vi "MCCPMTzero.vi"(8 "error in (no error)":errorcluster, 11 "MCCPMT in":refnum<class "MCCPMT.lvclass">) -> (0 "error out":errorcluster, 3 "MCCPMT out":refnum<class "MCCPMT.lvclass">)   [LabVIEW 2012, in "MCCPMT.lvclass"]
uses:
  MCCPMT.lvclass
  MCCPMT.lvclass/MCCPMT.ctl
  <vilib>/ULx/Create Channel.llb/ULx Create Channel (AO-Voltage-Basic).vi
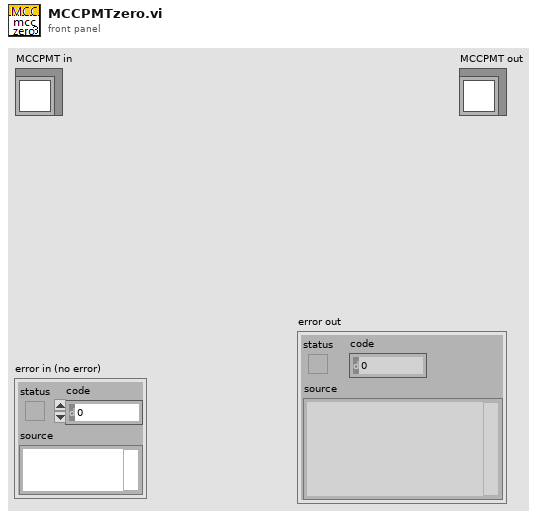
[diagram p1: front panel]
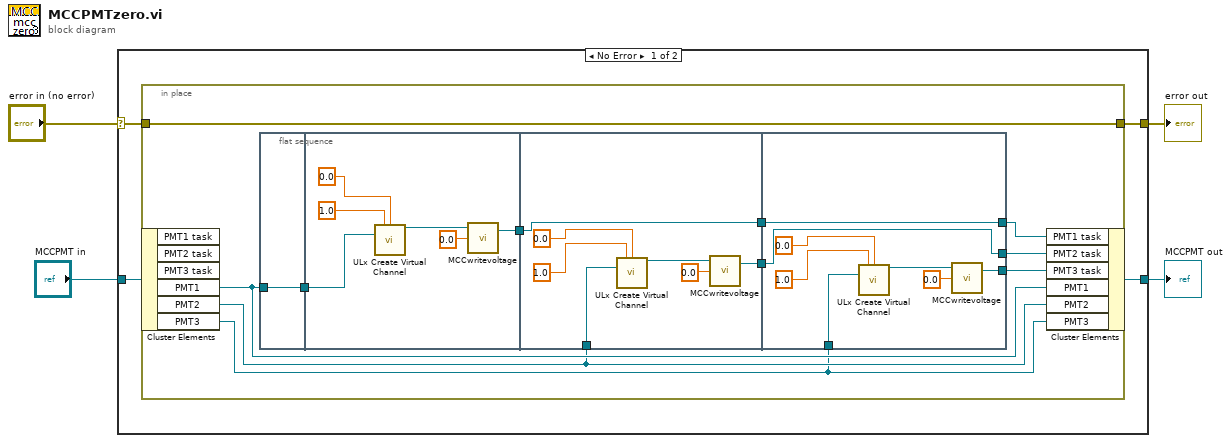
[diagram p0: block diagram]
diagram:
  n1 = case shown="No Error" "error in (no error)" {
    selector: "error in (no error)" -> [w6 w43]
    tunnel: [w5 w43] -> w3
    tunnel: [w7 w42] -> w1
    tunnel: "MCCPMT in" -> [w8 w42]
    frame No Error {
      n2 = in-place {
        in-place-border: w6 -> [w19]
        in-place-border: [w19] -> w5
        n3 = in-place-cluster #1(w8) -> ("PMT1"=w18:refnum<k21>, "PMT2"=w16:refnum<k21>, "PMT3"=w9:refnum<k21>)  [unwired: 3 out]
        n4 = flat-sequence {
          tunnel: w18 -> [w20]
          tunnel: [w20] -> w13
          tunnel: [w22] -> w17
          tunnel: w13 -> [w25]
          tunnel: w17 -> [w33]
          tunnel: w16 -> [w30]
          tunnel: [w33] -> w12
          tunnel: [w28] -> w11
          tunnel: [w40] -> w14
          tunnel: [w41] -> w15
          tunnel: w12 -> [w41]
          tunnel: w11 -> [w40]
          tunnel: w9 -> [w35]
          tunnel: [w34] -> w10
          frame #0 {
          }
          frame #1 {
            n5 = call-poly <vilib>:"ULx Create Virtual Channel.vi"("maximum value"=1.0, "minimum value"=0.0, "physical channels"=w25) -> ("task out"=w26:refnum<k24>)  [unwired: 11 in, 1 out]
            n6 = call "MCCwritevoltage.vi"("output voltage"=0.0, "task in"=w26) -> ("task out"=w22:refnum<k24>)  [unwired: 1 in, 1 out]
          }
          frame #2 {
            n7 = call-poly <vilib>:"ULx Create Virtual Channel.vi"("maximum value"=1.0, "minimum value"=0.0, "physical channels"=w30) -> ("task out"=w29:refnum<k24>)  [unwired: 11 in, 1 out]
            n8 = call "MCCwritevoltage.vi"("output voltage"=0.0, "task in"=w29) -> ("task out"=w28:refnum<k24>)  [unwired: 1 in, 1 out]
          }
          frame #3 {
            n9 = call-poly <vilib>:"ULx Create Virtual Channel.vi"("maximum value"=1.0, "minimum value"=0.0, "physical channels"=w35) -> ("task out"=w38:refnum<k24>)  [unwired: 11 in, 1 out]
            n10 = call "MCCwritevoltage.vi"("output voltage"=0.0, "task in"=w38) -> ("task out"=w34:refnum<k24>)  [unwired: 1 in, 1 out]
          }
        }
        n11 = in-place-cluster #1("PMT1 task"=w15, "PMT2 task"=w14, "PMT3 task"=w10, "PMT1"=w18, "PMT2"=w16, "PMT3"=w9) -> (w7:refnum<class "MCCPMT.lvclass">)
      }
    }
    frame Error {
    }
  }
  "error out" <- w3
  "MCCPMT out" <- w1
